vi "HelloWorld.vi"() -> ()   [LabVIEW 2023]
uses:
  <instrlib>/HandsOnPi2040/HandsOnPi2040.lvlib
  <instrlib>/HandsOnPi2040/Public/DigOuts.ctl
  <instrlib>/HandsOnPi2040/cti-drivers-lv-visa-main/CTI-Visa/Identity.ctl
  <instrlib>/HandsOnPi2040/cti-drivers-lv-visa-main/CTI-Visa/CTI-Visa.lvlib
panel:
  out "error out":errorcluster
  out "Identity":T1
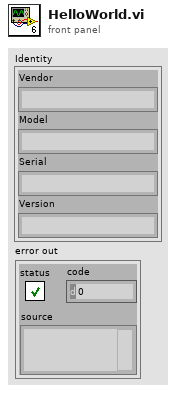
[diagram p1: front panel]
types:
  T1 = typedef "CTI-Visa.lvlib/Identity.ctl" = cluster{"Vendor":string, "Model":string, "Serial":string, "Version":string}
  T2 = typedef "HandsOnPi2040.lvlib/DigOuts.ctl" = enum16{"No DO - Error", "DO1 (GPIO2)", "DO2 (GPIO3)", "DO3 (GPIO4)", "DO4 (GPIO5)", "BEEP (GPIO6)"}
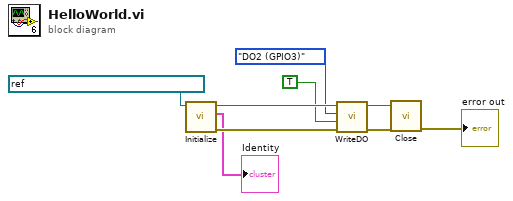
[diagram p0: block diagram]
diagram:
  n1 = call <instrlib>:"Initialize.vi"("VISA resource name"=refnum<visa-resource-name> "TCPIP0::10.0.2.15::6340::SOCKET") -> ("error out"=w9:errorcluster, "Identity"=→"Identity":T1, "VISA resource name out"=w8:refnum<visa-resource-name>)  [unwired: 8 in]
  n2 = call <instrlib>:"WriteDO.vi"("error in (no error)"=w9, "DO Value (True)"=TRUE, "Output"=DigOuts."DO2 (GPIO3)", "VISA resource name"=w8) -> ("error out"=w4:errorcluster, "VISA resource name out"=w3:refnum<visa-resource-name>)  [unwired: 6 in]
  n3 = call <instrlib>:"Close.vi"("error in (no error)"=w4, "VISA resource name"=w3) -> ("error out"=→"error out":errorcluster)  [unwired: 9 in]
